vi "Array_normalize.vi"(7 "Norm?":bool, 11 "Array":dbl[][](array[numeric]) format="%.4f") -> (3 "Array out":dbl[][](array[numeric]) format="%.4f")   [LabVIEW 2017]
panel:
  out "max index(es)":i32[](array[numeric])
  out "NaN/Path/Refnum?":bool[][](array[boolean])
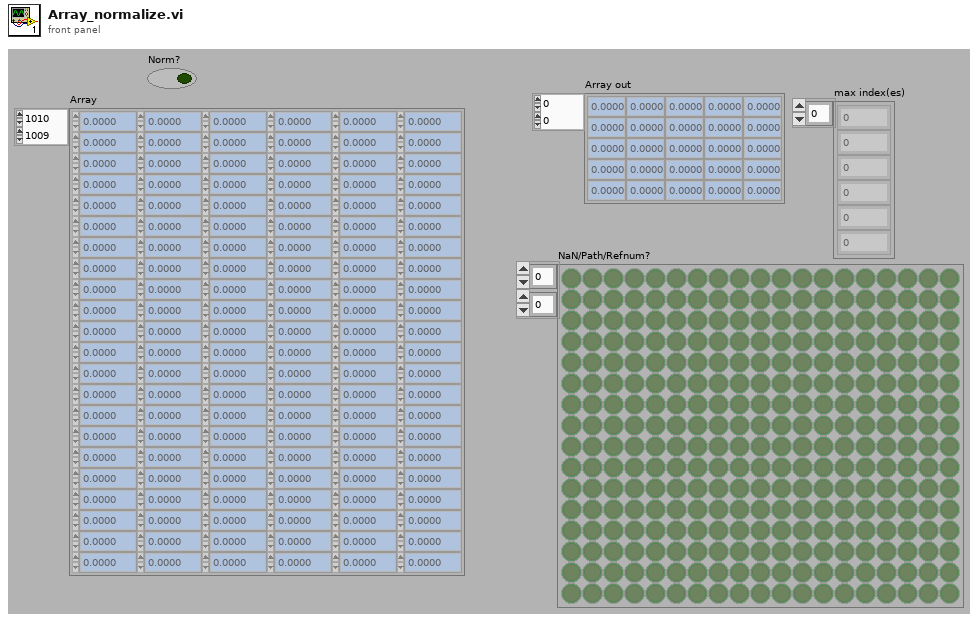
[diagram p1: front panel]
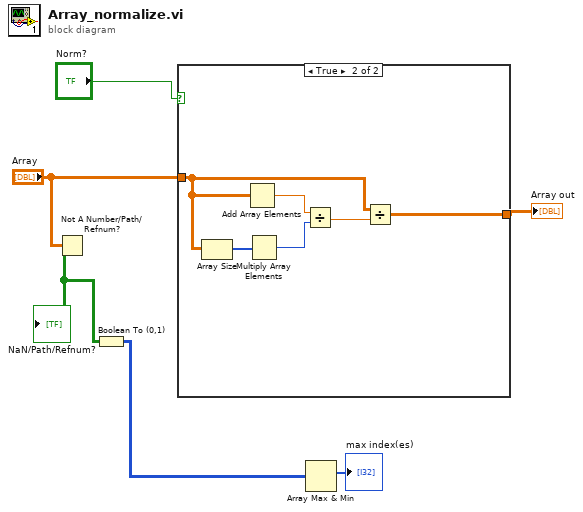
[diagram p0: block diagram]
diagram:
  n1 = Not A Number/Path/Refnum?(number/path/refnum="Array") -> (NaN/Path/Refnum?=w3:bool[][])
  "NaN/Path/Refnum?" <- w3
  n2 = Boolean To (0,1)(Boolean=w3) -> (0, 1=w2:i16[][])
  n3 = case shown="True" "Norm?" {
    tunnel: "Array" -> [w7 w9]
    tunnel: [w7 w8] -> w6
    frame False {
    }
    frame True {
      n4 = Array Size(array=w9) -> (size(s)=w13:i32[])
      n5 = Add Array Elements(numeric array=w9) -> (sum=w12:dbl)
      n6 = Multiply Array Elements(1:w13) -> (0:w11:i32)
      n7 = Divide(x=w12, y=w11) -> (x/y=w10:dbl)
      n8 = Divide(x=w9, y=w10) -> (x/y=w8:dbl[][])
    }
  }
  "Array out" <- w6
  n9 = Array Max & Min(array=w2) -> (max index (indices)=→"max index(es)":i32[])  [unwired: 3 out]
